vi "DEMO mmWave sequence execution.vi"() -> ()   [LabVIEW 2017]
uses:
  Classes/Sequence/SequenceSubvis/PolarizationSelect.ctl
  Classes/Sequence/SequenceSubvis/RF Direction.ctl
  Classes/Sequence/SequenceSubvis/PatchNewTestStep.ctl
  Classes/Datalog/DatalogSubvis/SearchableTag.ctl
  Classes/Datalog/DataLog.lvclass
panel:
  in  "Mode 1, 2, 3":i32=1
  out "i":i32
  in  "stop 2":bool
  out "Command":string
  out "Sweep Properties":T1
  out "NewSetup(postion)":T4
  in  "stop":bool
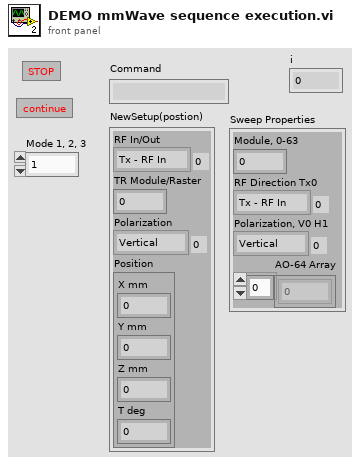
[diagram p1: front panel]
types:
  T1 = typedef "DataLog.lvclass/SearchableTag.ctl" = cluster{"Module, 0-63":i32, "RF Direction Tx0":T2, "Polarization, V0 H1":T3, "AO-64 Array":dbl[]}
  T2 = typedef "RF Direction.ctl" = enum16{"Tx - RF In", "Rx - RF Out"}
  T3 = typedef "PolarizationSelect.ctl" = enum16{"Vertical", "Horizontal"}
  T4 = typedef "PatchNewTestStep.ctl" = cluster{"RF In/Out":T2, "TR Module/Raster":i32, "Polarization":T3, "Position":cluster{"X mm":dbl, "Y mm":dbl, "Z mm":dbl, "T deg":dbl}}
  T5 = typedef "mWaveTestStep.ctl" = cluster{"StepType":T6, "RF In/Out":T2, "Module/Raster":i32, "Polarization":T3, "AO-64 Array":dbl[], "Position":cluster{"X mm":dbl, "Y mm":dbl, "Z mm":dbl, "T deg":dbl}}
  T6 = typedef "TestStepTypes.ctl" = enum16{"Patch", "Motion", "SweepTest", "RasterTest", "Finish", "64ModuleCfg"}
  T7 = cluster{"StepType":T6, "RF In/Out":T2, "Module/Raster":i32, "Polarization":T3, "AO-64 Array":dbl[], "Position":cluster{"X mm":dbl, "Y mm":dbl, "Z mm":dbl, "T deg":dbl}}[]
  T8 = cluster{"X mm":dbl, "Y mm":dbl, "Z mm":dbl, "T deg":dbl}
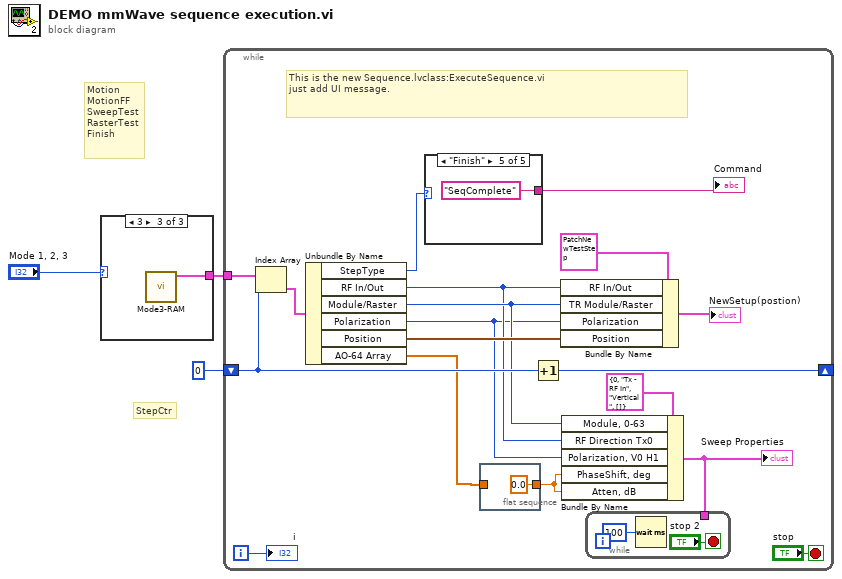
[diagram p0: block diagram]
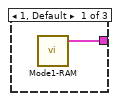
[diagram p2: hidden frame]
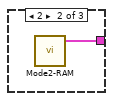
[diagram p3: hidden frame]
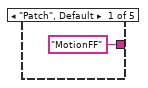
[diagram p4: hidden frame]
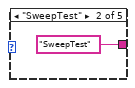
[diagram p5: hidden frame]
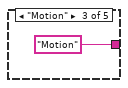
[diagram p6: hidden frame]
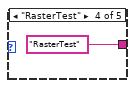
[diagram p7: hidden frame]
diagram:
  # "Motion\nMotionFF\nSweepTest\nRasterTest\nFinish"
  # "StepCtr"
  n1 = case shown="3" "Mode 1, 2, 3" {
    tunnel: [w4 w5 w6] -> w2
    frame 1, Default {
      n2 = call "Mode1-RAM.vi"() -> ("PAARD Super Mode"=w4:T5[])  [unwired: 11 in]
    }
    frame 2 {
      n3 = call "Mode2-RAM.vi"() -> ("PAARD Super Mode"=w5:T7)  [unwired: 11 in]
    }
    frame 3 {
      n4 = call "Mode3-RAM.vi"() -> ("PAARD Super Mode"=w6:T7)  [unwired: 11 in]
    }
  }
  n5 = while {
    shift-right: [w15] -> _
    shift-left: 0 -> [w16]
    tunnel: w2 -> [w23]
    i -> [w20]
    stop <- "stop" stop-if-true
    # "This is the new Sequence.lvclass:ExecuteSequence.vi\njust add UI message."
    n6 = Index Array(array=w23, index=w16) -> (element=w18:T5)
    n7 = Unbundle By Name(w18) -> ("StepType"=w8:T6, "RF In/Out"=w12:T2, "Module/Raster"=w13:i32, "Polarization"=w11:T3, "Position"=w17:T8, "AO-64 Array"=w10:dbl[])
    n8 = case shown="\"Finish\"" w8 {
      tunnel: ["MotionFF" ("Command") "SweepTest" ("Command") "Motion" ("Command") "RasterTest" ("Command") "SeqComplete" ("Command")] -> w7
      frame "Patch", Default {
      }
      frame "SweepTest" {
      }
      frame "Motion" {
      }
      frame "RasterTest" {
      }
      frame "Finish" {
      }
    }
    "Command" <- w7
    n9 = flat-sequence {
      tunnel: w10 -> [_]
      tunnel: [0.0 ("PhaseShift, deg")] -> w9
      frame #0 {
      }
    }
    n10 = Increment(x=w16) -> (x+1=w15:i32)
    n11 = Bundle By Name(cluster=T4 {"RF In/Out"=enum."Tx - RF In", "TR Module/Raster"=0, "Polarization"=enum."Vertical", "Position"={"X mm"=0.0, "Y mm"=0.0, "Z mm"=0.0, "T deg"=0.0}} ("NewSetup"), "RF In/Out"=w12, "TR Module/Raster"=w13, "Polarization"=w11, "Position"=w17) -> (→"NewSetup(postion)":T4)
    n12 = Bundle By Name(cluster=T1 {"Module, 0-63"=0, "RF Direction Tx0"=enum."Tx - RF In", "Polarization, V0 H1"=enum."Vertical", "AO-64 Array"=[]} ("SweepProperties"), "Module, 0-63"=w13, "RF Direction Tx0"=w12, "Polarization, V0 H1"=w11, "PhaseShift, deg"=w9, "Atten, dB"=w9) -> (w21:T1)
    "Sweep Properties" <- w21
    n13 = while {
      tunnel: w21 -> [_]
      stop <- "stop 2" stop-if-true
      n14 = Wait (ms)(milliseconds to wait=u32 100) -> ()  [unwired: 1 out]
    }
    "i" <- w20
  }
